vi "_test fade.vi"() -> ()   [LabVIEW 2012]
uses:
  Fading/_fadetype.ctl
panel:
  in  "Fade time (ms)":i32=250
  in  "Set":bool
  in  "Fade (Exponential)":T1
  out "Transparency (%)":u8 max=100 step=1
  in  "Target":u8 max=100 step=1
  in  "fade":bool
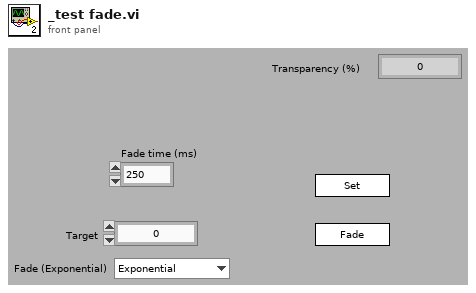
[diagram p1: front panel]
types:
  T1 = typedef "_fadetype.ctl" = enum16{"Exponential", "Linear"}
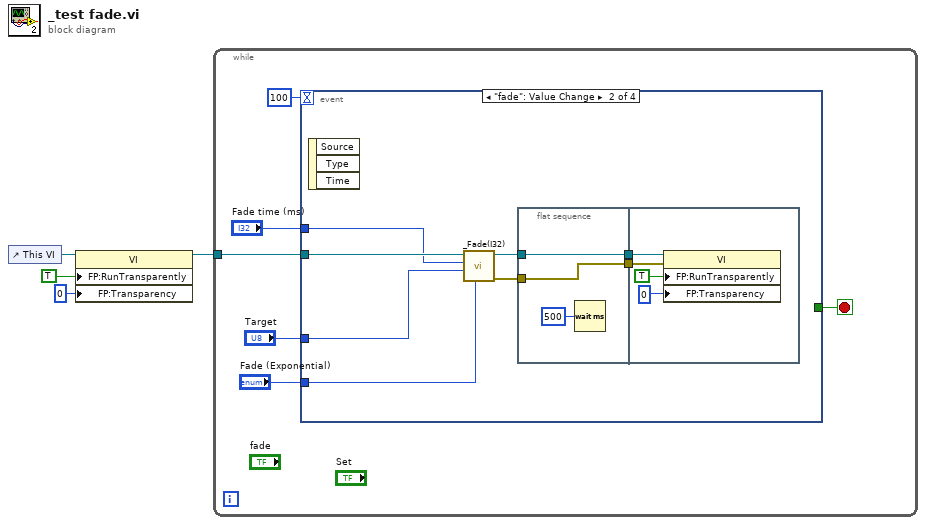
[diagram p0: block diagram]
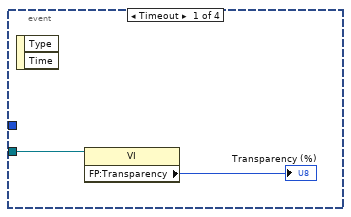
[diagram p2: hidden frame]
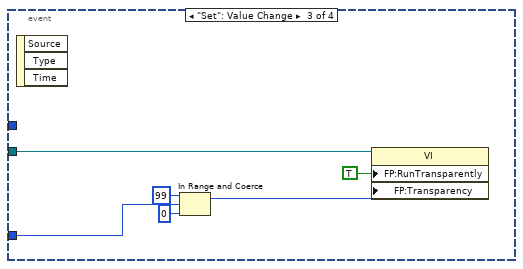
[diagram p3: hidden frame]
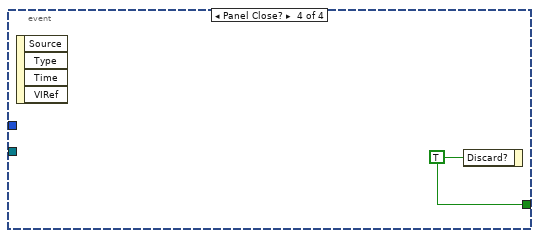
[diagram p4: hidden frame]
diagram:
  n1 = control-ref of="This VI"() -> (w4:refnum<vi>)
  n2 = property class="VI"(reference=w4, "FP:RunTransparently"=TRUE ("Front Panel Window:Run VI Transparently"), "FP:Transparency"=u8 0 ("Front Panel Window:Transparency")) -> (reference out=w3:refnum<vi>)  [unwired: 1 in, 1 out]
  n3 = while {
    tunnel: w3 -> [w8]
    stop <- w9 stop-if-true
    n4 = event shown="[1] \"fade\": Value Change" {
      selector: _ -> [_ _ _ _]
      dyn-events: _ -> [_ _ _ _]
      timeout: 100 -> [_ _ _ _]
      tunnel: [_ _ _ w34] -> w9
      tunnel: w8 -> [w12 w14 w32 _]
      tunnel: "Target" -> [_ w20 w31 _]
      tunnel: "Fade (Exponential)" -> [_ w19 _ _]
      tunnel: "Fade time (ms)" -> [_ w13 _ _]
      event Timeout {
        n5 = event-data() -> ()  [unwired: 3 out]
        n6 = property class="VI"(reference=w12) -> ("FP:Transparency"=→"Transparency (%)":u8)  [unwired: 1 in, 2 out]
      }
      event "fade": Value Change {
        n7 = event-data() -> ()  [unwired: 4 out]
        n8 = call "_Fade(I32).vi"("Fade (Exponential)"=w19, "Target Transparency (0)"=w20, "Fade time (ms)"=w13, "VI Reference (calling VI)"=w14) -> ("error out"=w17:errorcluster, "dup VI Reference"=w18:refnum<vi>)  [unwired: 1 in, 5 out]
        n9 = flat-sequence {
          tunnel: w18 -> [w22]
          tunnel: w17 -> [w21]
          tunnel: [w22] -> w16
          tunnel: [w21] -> w15
          tunnel: w16 -> [w27]
          tunnel: w15 -> [w26]
          frame #0 {
            n10 = Wait (ms)(milliseconds to wait=u32 500) -> ()  [unwired: 1 out]
          }
          frame #1 {
            n11 = property class="VI"(reference=w27, error in=w26, "FP:RunTransparently"=TRUE ("Front Panel Window:Run VI Transparently"), "FP:Transparency"=u8 0 ("Front Panel Window:Transparency")) -> ()  [unwired: 2 out]
          }
        }
      }
      event "Set": Value Change {
        n12 = event-data() -> ()  [unwired: 4 out]
        n13 = In Range and Coerce(upper limit=u8 99, x=w31, lower limit=u8 0) -> (coerced(x)=w28:u8)  [unwired: 1 out]
        n14 = property class="VI"(reference=w32, "FP:RunTransparently"=TRUE ("Front Panel Window:Run VI Transparently"), "FP:Transparency"=w28) -> ()  [unwired: 1 in, 2 out]
      }
      event Panel Close? {
        w34 = TRUE ("Discard?")
        n15 = event-data() -> ()  [unwired: 5 out]
        n16 = event-data("Discard?"=w34) -> ()  [unwired: 1 in, 1 out]
      }
    }
  }
